vi "BSA_F600_Dantec_Example.vi"() -> ()   [LabVIEW 2018]
panel:
  in  "BSACtrl.IBSA 2":refnum<k7>
  in  "configuration":i32
  in  "processor":i32
  out "error out":errorcluster {"code" format="%.0x"}
  out "GetConnectState":i32
  out "Data":T1(graph)
  in  "Show Data":bool
  in  "Stop Acq":bool
  in  "Start ACQ":bool
  in  "Processor Properties:":i32(listbox)
  in  "Get Properties":bool
  in  "Disconnect":bool
  in  "Property value":string
  in  "Change value":bool
  in  "Connect state":bool
  in  "IP adress":string="10.10.100.130"
  in  "Connect IP":bool
  in  "Set Processor Properties:":i32(listbox) caption="Property"
  in  "stop":bool
  # "LabVIEW example for the BSA.Ctrl for the BSA Processor."
  # "IP - Adress:"
  # "Property value:"
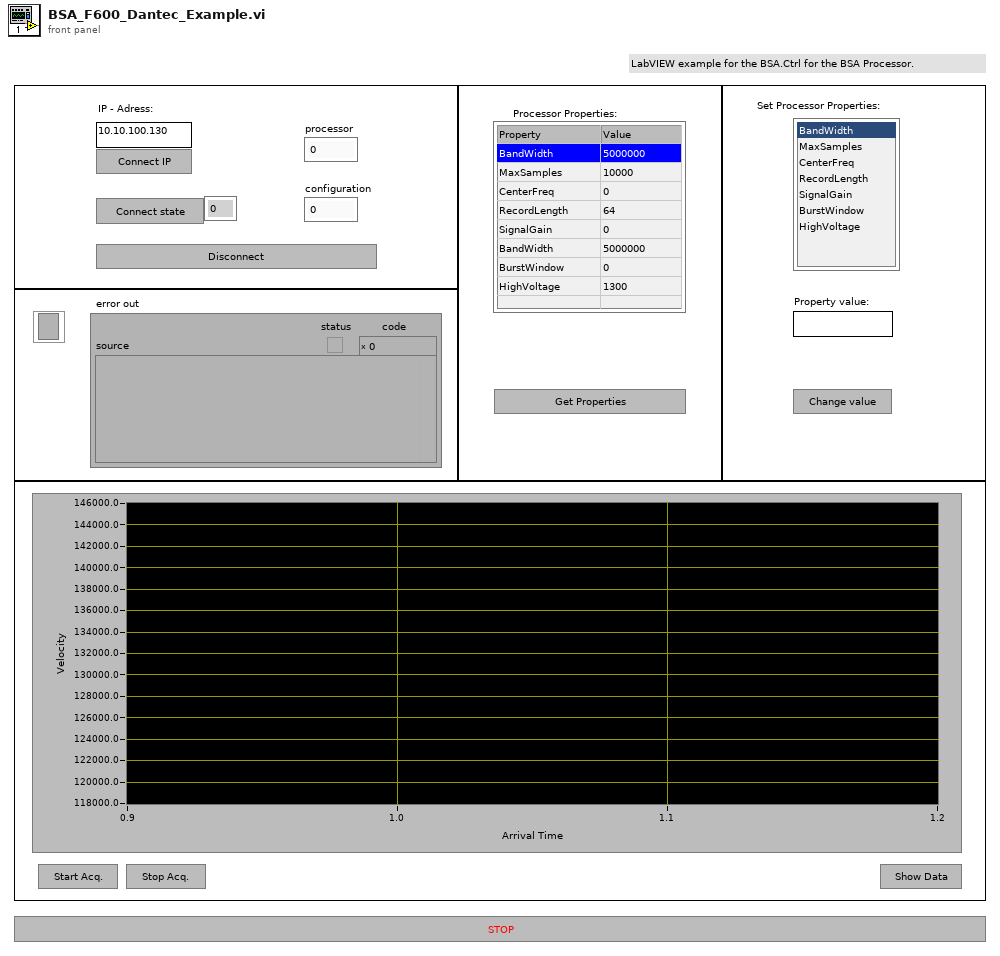
[diagram p1: front panel]
types:
  T1 = cluster{"Array Constant":dbl[], "Array Constant":dbl[]}
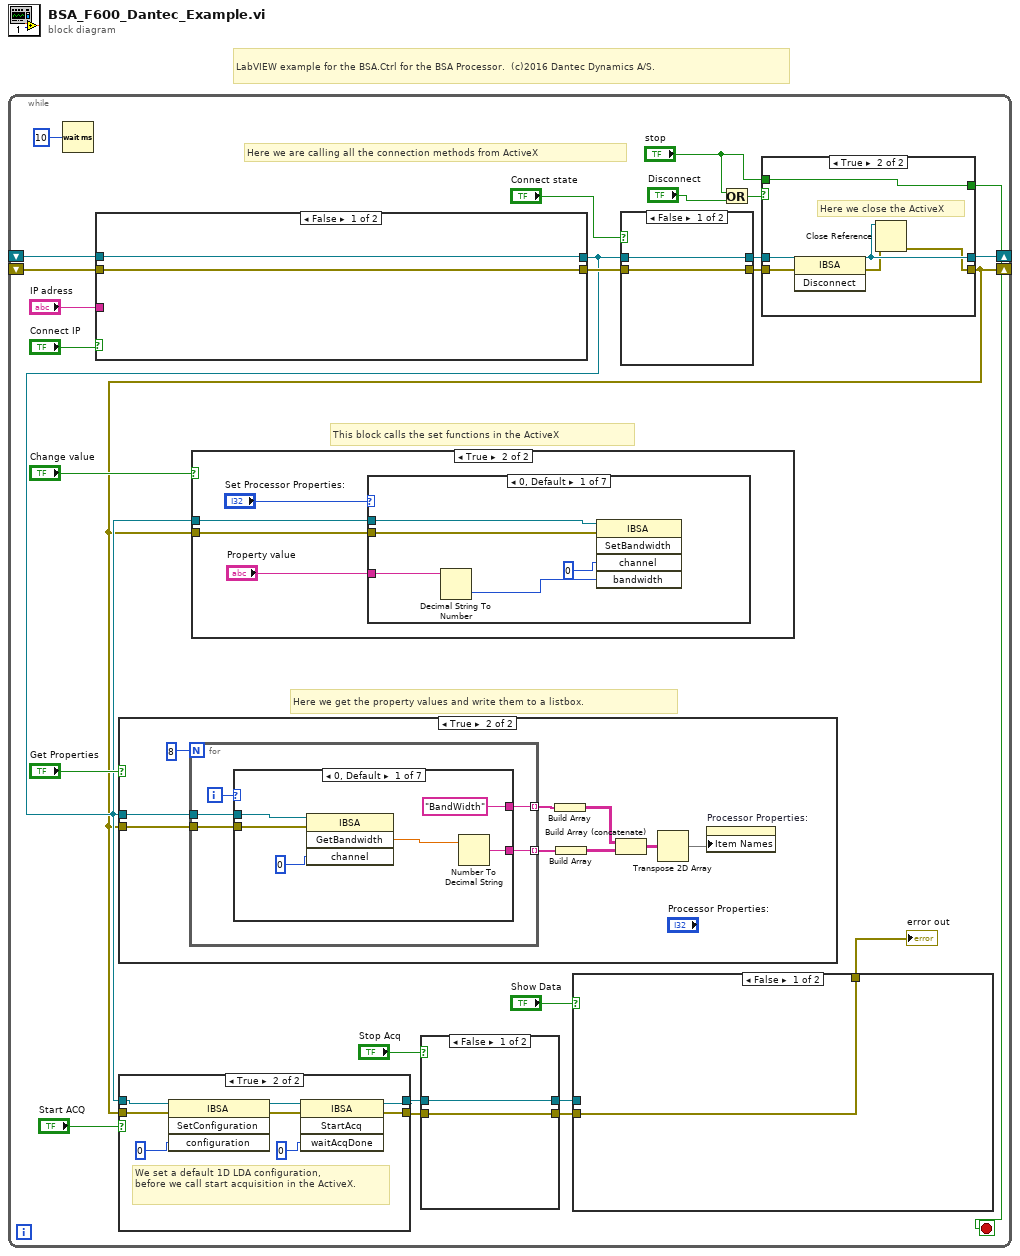
[diagram p0: block diagram]
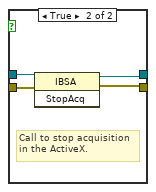
[diagram p3: hidden frame]
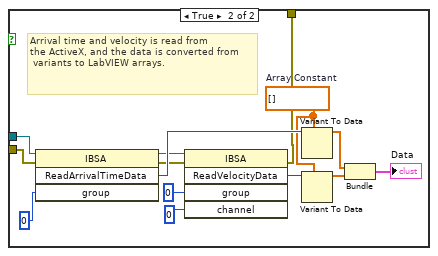
[diagram p4: hidden frame]
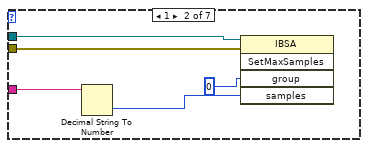
[diagram p6: hidden frame]
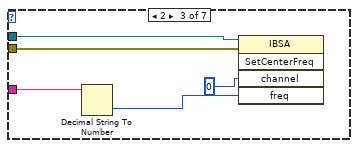
[diagram p7: hidden frame]
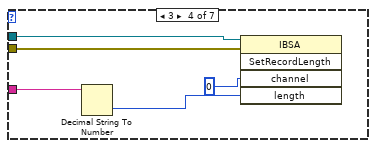
[diagram p8: hidden frame]
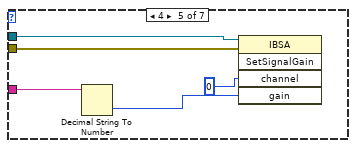
[diagram p9: hidden frame]
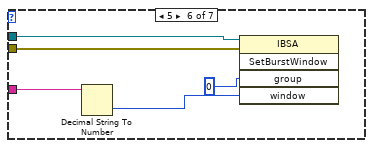
[diagram p10: hidden frame]
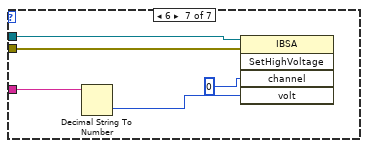
[diagram p11: hidden frame]
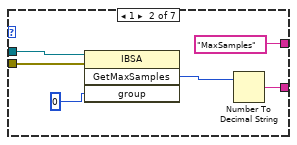
[diagram p13: hidden frame]
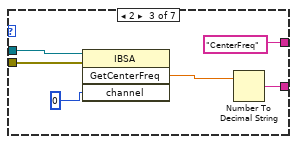
[diagram p14: hidden frame]
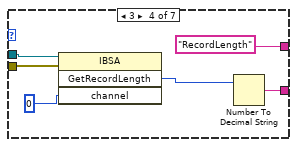
[diagram p15: hidden frame]
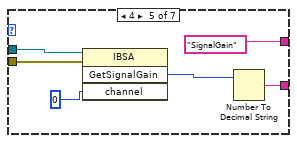
[diagram p16: hidden frame]
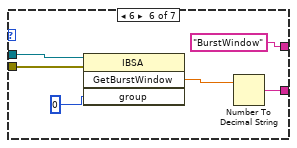
[diagram p17: hidden frame]
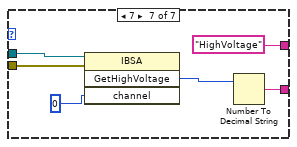
[diagram p18: hidden frame]
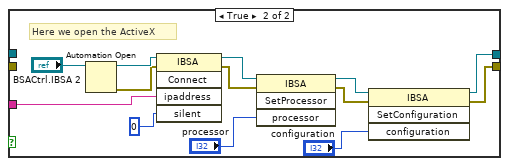
[diagram p19: hidden frame]
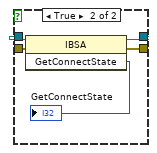
[diagram p20: hidden frame]
diagram:
  # "LabVIEW example for the BSA.Ctrl for the BSA Processor.  (c)2016 Dantec Dynamics A/S."
  n1 = while {
    shift-right: [w7] -> _
    shift-left: _ -> [w6]
    shift-right: [w2] -> _
    shift-left: _ -> [w5]
    stop <- w8 stop-if-true
    # "Here we get the property values and write them to a listbox."
    # "This block calls the set functions in the ActiveX"
    # "Here we are calling all the connection methods from ActiveX"
    n2 = Wait (ms)(milliseconds to wait=u32 10) -> ()  [unwired: 1 out]
    n3 = case shown="False" "Connect IP" {
      tunnel: [w154 w162] -> w3
      tunnel: [w153 w160] -> w4
      tunnel: "IP adress" -> [_ w166]
      tunnel: w6 -> [w154 _]
      tunnel: w5 -> [w153 _]
      frame False {
      }
      frame True {
        # "Here we open the ActiveX"
        n4 = Automation Open(Automation Refnum="BSACtrl.IBSA 2") -> (Automation Refnum=w156:refnum<k7>, error out=w155:errorcluster)  [unwired: 3 in]
        n5 = invoke class="IBSA" method="Connect"(reference=w156, error in=w155, "ipaddress"=w166, "silent"=0) -> (reference out=w165:refnum<k7>, error out=w164:errorcluster)  [unwired: 1 in, 3 out]
        n6 = invoke class="IBSA" method="SetProcessor"(reference=w165, error in=w164, "processor"="processor") -> (reference out=w163:refnum<k7>, error out=w161:errorcluster)  [unwired: 1 in, 2 out]
        n7 = invoke class="IBSA" method="SetConfiguration"(reference=w163, error in=w161, "configuration"="configuration") -> (reference out=w162:refnum<k7>, error out=w160:errorcluster)  [unwired: 1 in, 2 out]
      }
    }
    n8 = case shown="False" "Connect state" {
      tunnel: w3 -> [w169 w174]
      tunnel: [w169 w173] -> w21
      tunnel: w4 -> [w168 w172]
      tunnel: [w168 w171] -> w22
      frame False {
      }
      frame True {
        n9 = invoke class="IBSA" method="GetConnectState"(reference=w174, error in=w172) -> (reference out=w173:refnum<k7>, error out=w171:errorcluster, "GetConnectState"=→"GetConnectState":i32)  [unwired: 1 in]
      }
    }
    n10 = Or(x="stop", y="Disconnect") -> (x .or. y?=w11:bool)
    n11 = case shown="True" w11 {
      tunnel: w21 -> [w176 w183]
      tunnel: w22 -> [w177 w182]
      tunnel: [w177 w178] -> w2
      tunnel: [w176 w181] -> w7
      tunnel: "stop" -> [_ w179]
      tunnel: [FALSE ("stop") w179] -> w8
      frame False {
      }
      frame True {
        # "Here we close the ActiveX"
        n12 = invoke class="IBSA" method="Disconnect"(reference=w183, error in=w182) -> (reference out=w181:refnum<k7>, error out=w180:errorcluster)  [unwired: 1 in, 1 out]
        n13 = Close Reference(reference=w181, error in (no error)=w180) -> (error out=w178:errorcluster)
      }
    }
    n14 = case shown="True" "Get Properties" {
      tunnel: w3 -> [_ w99]
      tunnel: w2 -> [_ w98]
      frame False {
      }
      frame True {
        n15 = for {
          N: 8 -> [_]
          tunnel: [w109] -> w101 mode=indexing
          tunnel: w99 -> [w108]
          tunnel: w98 -> [w107]
          tunnel: [w106] -> w97 mode=indexing
          i -> [w110]
          n16 = case shown="0, Default" w110 {
            tunnel: [w114 w121 w126 w132 w138 w145 w152] -> w109
            tunnel: w108 -> [w112 w119 w124 w130 w137 w143 w148]
            tunnel: w107 -> [w113 w118 w125 w131 w136 w142 w149]
            tunnel: ["BandWidth" "MaxSamples" "CenterFreq" "RecordLength" "SignalGain" "BurstWindow" "HighVoltage"] -> w106
            frame 0, Default {
              n17 = invoke class="IBSA" method="GetBandwidth"(reference=w112, error in=w113, "channel"=0) -> ("GetBandwidth"=w115:sgl)  [unwired: 1 in, 3 out]
              n18 = Number To Decimal String(number=w115) -> (decimal integer string=w114:string)  [unwired: 1 in]
            }
            frame 1 {
              n19 = invoke class="IBSA" method="GetMaxSamples"(reference=w119, error in=w118, "group"=0) -> ("GetMaxSamples"=w122:i32)  [unwired: 1 in, 3 out]
              n20 = Number To Decimal String(number=w122) -> (decimal integer string=w121:string)  [unwired: 1 in]
            }
            frame 2 {
              n21 = invoke class="IBSA" method="GetCenterFreq"(reference=w124, error in=w125, "channel"=0) -> ("GetCenterFreq"=w127:sgl)  [unwired: 1 in, 3 out]
              n22 = Number To Decimal String(number=w127) -> (decimal integer string=w126:string)  [unwired: 1 in]
            }
            frame 3 {
              n23 = invoke class="IBSA" method="GetRecordLength"(reference=w130, error in=w131, "channel"=0) -> ("GetRecordLength"=w133:i32)  [unwired: 1 in, 3 out]
              n24 = Number To Decimal String(number=w133) -> (decimal integer string=w132:string)  [unwired: 1 in]
            }
            frame 4 {
              n25 = invoke class="IBSA" method="GetSignalGain"(reference=w137, error in=w136, "channel"=0) -> ("GetSignalGain"=w139:i32)  [unwired: 1 in, 3 out]
              n26 = Number To Decimal String(number=w139) -> (decimal integer string=w138:string)  [unwired: 1 in]
            }
            frame 6 {
              n27 = invoke class="IBSA" method="GetBurstWindow"(reference=w143, error in=w142, "group"=0) -> ("GetBurstWindow"=w146:sgl)  [unwired: 1 in, 3 out]
              n28 = Number To Decimal String(number=w146) -> (decimal integer string=w145:string)  [unwired: 1 in]
            }
            frame 7 {
              n29 = invoke class="IBSA" method="GetHighVoltage"(reference=w148, error in=w149, "channel"=0 ("group")) -> ("GetHighVoltage"=w150:i32)  [unwired: 1 in, 3 out]
              n30 = Number To Decimal String(number=w150) -> (decimal integer string=w152:string)  [unwired: 1 in]
            }
          }
        }
        n31 = Build Array(w97) -> (w104:string[][])
        n32 = Build Array(w101) -> (w103:string[][])
        n33 = Build Array (concatenate)(w104, w103) -> (w102:string[][])
        n34 = Transpose 2D Array(2D array=w102) -> (transposed array=w105:string[][])
        n35 = property on="Processor Properties:" class="MCListbox (strict)"("Item Names"=w105) -> ()  [unwired: 2 in, 2 out]
      }
    }
    n36 = case shown="True" "Start ACQ" {
      tunnel: [w28 w32] -> w15
      tunnel: [w27 w31] -> w16
      tunnel: w3 -> [w28 w30]
      tunnel: w2 -> [w27 w29]
      frame False {
      }
      frame True {
        # "We set a default 1D LDA configuration,\nbefore we call start acquisition in the ActiveX."
        n37 = invoke class="IBSA" method="SetConfiguration"(reference=w30, error in=w29, "configuration"=0 ("config")) -> (reference out=w35:refnum<k7>, error out=w34:errorcluster)  [unwired: 1 in, 2 out]
        n38 = invoke class="IBSA" method="StartAcq"(reference=w35, error in=w34, "waitAcqDone"=0) -> (reference out=w32:refnum<k7>, error out=w31:errorcluster)  [unwired: 1 in, 2 out]
      }
    }
    n39 = case shown="True" "Change value" {
      tunnel: w2 -> [_ w59]
      tunnel: w3 -> [_ w58]
      frame False {
      }
      frame True {
        n40 = case shown="0, Default" "Set Processor Properties:" {
          tunnel: "Property value" -> [w66 w71 w76 w81 w86 w91 w96]
          tunnel: w59 -> [w65 w68 w75 w80 w85 w88 w95]
          tunnel: w58 -> [w64 w67 w74 w79 w84 w87 w94]
          frame 0, Default {
            n41 = Decimal String To Number(string=w66) -> (number=w63:i32)  [unwired: 2 in, 1 out]
            n42 = invoke class="IBSA" method="SetBandwidth"(reference=w64, error in=w65, "channel"=0, "bandwidth"=w63) -> ()  [unwired: 1 in, 5 out]
          }
          frame 1 {
            n43 = Decimal String To Number(string=w71) -> (number=w70:i32)  [unwired: 2 in, 1 out]
            n44 = invoke class="IBSA" method="SetMaxSamples"(reference=w67, error in=w68, "group"=0, "samples"=w70) -> ()  [unwired: 1 in, 5 out]
          }
          frame 2 {
            n45 = Decimal String To Number(string=w76) -> (number=w73:i32)  [unwired: 2 in, 1 out]
            n46 = invoke class="IBSA" method="SetCenterFreq"(reference=w74, error in=w75, "channel"=0, "freq"=w73) -> ()  [unwired: 1 in, 5 out]
          }
          frame 3 {
            n47 = Decimal String To Number(string=w81) -> (number=w78:i32)  [unwired: 2 in, 1 out]
            n48 = invoke class="IBSA" method="SetRecordLength"(reference=w79, error in=w80, "channel"=0, "length"=w78) -> ()  [unwired: 1 in, 5 out]
          }
          frame 4 {
            n49 = Decimal String To Number(string=w86) -> (number=w82:i32)  [unwired: 2 in, 1 out]
            n50 = invoke class="IBSA" method="SetSignalGain"(reference=w84, error in=w85, "channel"=0, "gain"=w82) -> ()  [unwired: 1 in, 5 out]
          }
          frame 5 {
            n51 = Decimal String To Number(string=w91) -> (number=w90:i32)  [unwired: 2 in, 1 out]
            n52 = invoke class="IBSA" method="SetBurstWindow"(reference=w87, error in=w88, "group"=0, "window"=w90) -> ()  [unwired: 1 in, 5 out]
          }
          frame 6 {
            n53 = Decimal String To Number(string=w96) -> (number=w92:i32)  [unwired: 2 in, 1 out]
            n54 = invoke class="IBSA" method="SetHighVoltage"(reference=w94, error in=w95, "channel"=0 ("group"), "volt"=w92) -> ()  [unwired: 1 in, 5 out]
          }
        }
      }
    }
    n55 = case shown="False" "Stop Acq" {
      tunnel: w15 -> [w38 w42]
      tunnel: w16 -> [w37 w41]
      tunnel: [w38 w40] -> w17
      tunnel: [w37 w39] -> w18
      frame False {
      }
      frame True {
        # "Call to stop acquisition\nin the ActiveX."
        n56 = invoke class="IBSA" method="StopAcq"(reference=w42, error in=w41) -> (reference out=w40:refnum<k7>, error out=w39:errorcluster)  [unwired: 1 in, 1 out]
      }
    }
    n57 = case shown="False" "Show Data" {
      tunnel: w17 -> [_ w47]
      tunnel: w18 -> [w43 w46]
      tunnel: [w43 w44] -> w1
      frame False {
      }
      frame True {
        w45 = dbl[] []  # Array Constant
        # "Arrival time and velocity is read from \nthe ActiveX, and the data is converted from\n variants to LabVIEW arrays."
        n58 = invoke class="IBSA" method="ReadArrivalTimeData"(reference=w47, error in=w46, "group"=0) -> (reference out=w49:refnum<k7>, error out=w48:errorcluster, "ReadArrivalTimeData"=w57:variant)  [unwired: 1 in, 1 out]
        n59 = invoke class="IBSA" method="ReadVelocityData"(reference=w49, error in=w48, "group"=0, "channel"=0 ("ich")) -> (error out=w44:errorcluster, "ReadVelocityData"=w56:variant)  [unwired: 1 in, 3 out]
        n60 = Variant To Data(type=w45, Variant=w57) -> (data=w53:dbl[])  [unwired: 1 in, 1 out]
        n61 = Variant To Data(type=w45, Variant=w56) -> (data=w55:dbl[])  [unwired: 1 in, 1 out]
        n62 = Bundle "Bundle"("Array Constant"=w53, "Array Constant"=w55) -> (→"Data":T1)  [unwired: 1 in]
      }
    }
    "error out" <- w1
  }
